vi "Connector 0 AO Engine Sim.vi"(0 "Packets":u64[](array[numeric])=[0, 0]) -> ()   [LabVIEW 2014]
uses:
  <vilib>/rvi/eio/common/nirviEmuTemplateMethod_errors.vi
  <vilib>/eio/EIONode/EIONode.xnode
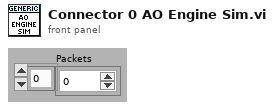
[diagram p1: front panel]
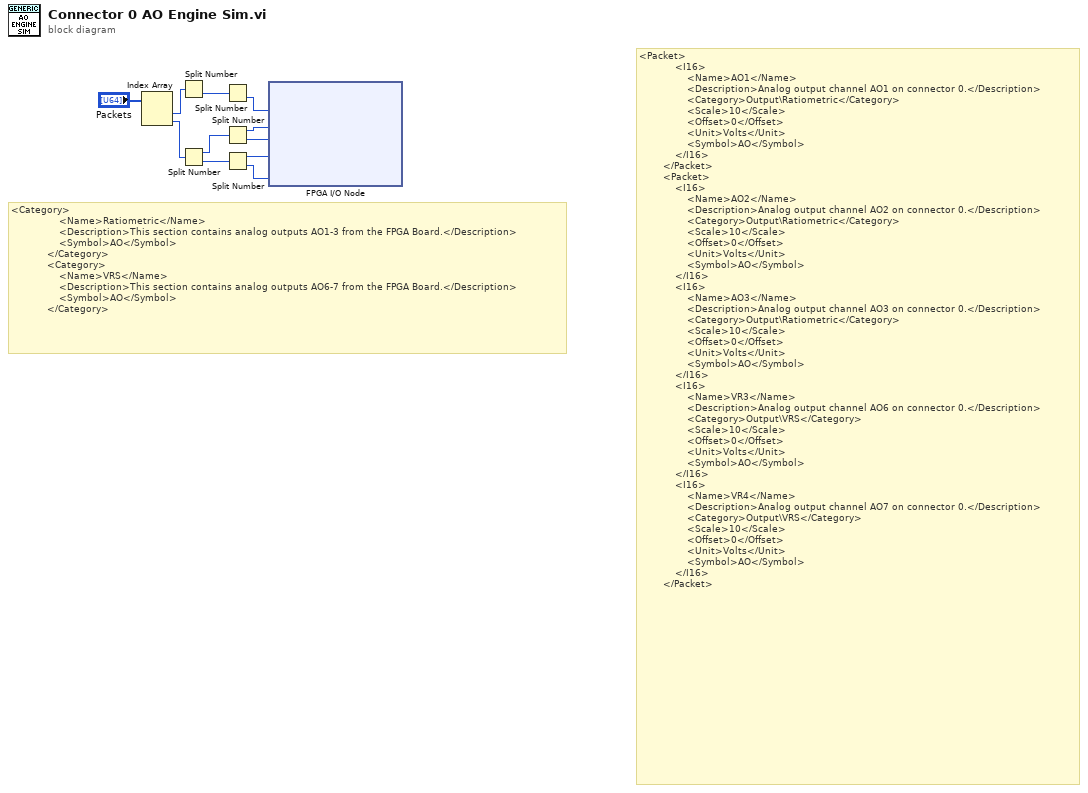
[diagram p0: block diagram]
diagram:
  # "<Category>\n                <Name>Ratiometric</Name>\n                <Description>This section contains analog outputs AO1-3 from the FPGA Board.</Description>\n                <Symbol>AO</Symbol>\n            </Category>\n            <Category>\n                <Name>VRS</Name>\n                <Description>This section contains analog outputs AO6-7 from the FPGA Board.</Description>\n                <Symbol>AO</Symbol>\n            </Category>"
  # "<Packet>\n            <I16>\n                <Name>AO1</Name>\n                <Description>Analog output channel AO1 on connector 0.</Description>\n                <Category>Output\\Ratiometric</Category>\n                <Scale>10</Scale>\n                <Offset>0</Offset>\n                <Unit>Volts</Unit>\n                <Symbol>AO</Symbol>\n            </I16>\n        </Packet>\n        <Packet>\n            <I16>\n                <Name>AO2</Name>\n                <Description>Analog output channel AO2 on connector 0.</Description>\n                <Category>Output\\Ratiometric</Category>\n                <Scale>10</Scale>\n                <Offset>0</Offset>\n                <Unit>Volts</Unit>\n                <Symbol>AO</Symbol>\n            </I16>\n            <I16>\n                <Name>AO3</Name>\n                <Description>Analog output channel AO3 on connector 0.</Description>\n                <Category>Output\\Ratiometric</Category>\n                <Scale>10</Scale>\n                <Offset>0</Offset>\n                <Unit>Volts</Unit>\n                <Symbol>AO</Symbol>\n            </I16>\n            <I16>\n                <Name>VR3</Name>\n                <Description>Analog output channel AO6 on connector 0.</Description>\n                <Category>Output\\VRS</Category>\n                <Scale>10</Scale>\n                <Offset>0</Offset>\n                <Unit>Volts</Unit>\n                <Symbol>AO</Symbol>\n            </I16>\n            <I16>\n                <Name>VR4</Name>\n                <Description>Analog output channel AO7 on connector 0.</Description>\n                <Category>Output\\VRS</Category>\n                <Scale>10</Scale>\n                <Offset>0</Offset>\n                <Unit>Volts</Unit>\n                <Symbol>AO</Symbol>\n            </I16>\n        </Packet>"
  n1 = Index Array(array="Packets") -> (element #1=w10:u64, element #2=w11:u64)  [unwired: 2 in]
  n2 = Split Number(x=w10) -> (lo(x)=w3:u32)  [unwired: 1 out]
  n3 = Split Number(x=w11) -> (hi(x)=w2:u32, lo(x)=w1:u32)
  n4 = Split Number(x=w3) -> (lo(x)=w8:u16)  [unwired: 1 out]
  n5 = Split Number(x=w2) -> (hi(x)=w7:u16, lo(x)=w6:u16)
  n6 = Split Number(x=w1) -> (hi(x)=w5:u16, lo(x)=w4:u16)
  n7 = xnode "FPGA I/O Node"("Connector0/AO1"=w8, "Connector0/AO7"=w7, "Connector0/AO6"=w6, "Connector0/AO3"=w5, "Connector0/AO2"=w4) -> ()  [unwired: 5 in, 5 out]
